vi "Configure Measurement (Period).vi"(7 "Frequency Resolution (100E-9s)":dbl=1e-07 format="%^#_7g", 8 "error in (no error)":errorcluster, 9 "Period Estimate (100E-9s)":dbl=1e-07 format="%^#_7g", 10 "Channel (1:Channel 1)":i32(ring)=1 items=["Channel 1"=1, "Channel 2"=2, "Channel 3"=3], 11 "VISA resource name":refnum<visa-resource-name>) -> (0 "error out":errorcluster, 3 "VISA resource name out":refnum<visa-resource-name>)   [LabVIEW 2024, in "Agilent 532XX Series.lvlib"]
doc: "Configures the parameters required for Period measurements."
uses:
  Agilent 532XX Series.lvlib
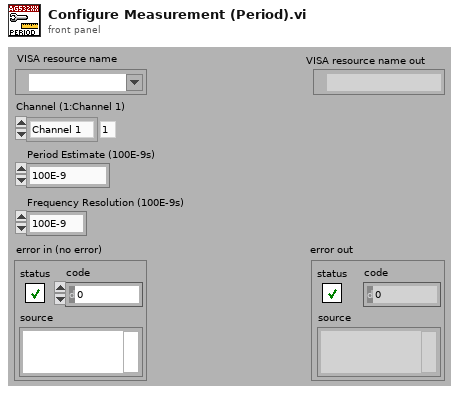
[diagram p1: front panel]
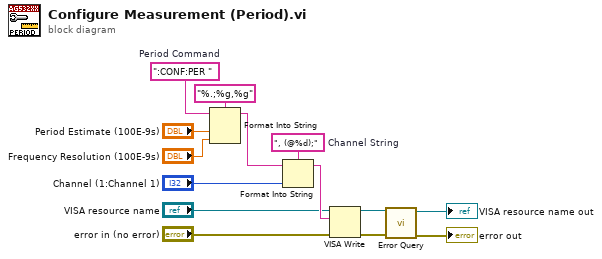
[diagram p0: block diagram]
diagram:
  w13 = ", (@%d);"  # Channel String
  w2 = ":CONF:PER "  # Period Command
  n1 = Format Into String(format string="%.;%g,%g", initial string=w2, "Period Estimate (100E-9s)", "Frequency Resolution (100E-9s)") -> (resulting string=w3:string)  [unwired: 1 in, 1 out]
  n2 = Format Into String(format string=w13, initial string=w3, "Channel (1:Channel 1)") -> (resulting string=w10:string)  [unwired: 1 in, 1 out]
  n3 = VISA Write(VISA resource name="VISA resource name", write buffer=w10, error in (no error)="error in (no error)") -> (VISA resource name out=w12:refnum<visa-resource-name>, error out=w11:errorcluster)  [unwired: 1 out]
  n4 = call "Error Query.vi"("error in (no error)"=w11, "VISA resource name"=w12) -> ("error out"=→"error out":errorcluster, "VISA resource name out"=→"VISA resource name out":refnum<visa-resource-name>)  [unwired: 8 out]
